vi "Read Format String.vi"(9 "NumericText in":refnum<class "NumericText.lvclass">) -> (3 "NumericText out":refnum<class "NumericText.lvclass">, 4 "Format String":string)   [LabVIEW 2014, in "Raspberry Pi Compatible Compiler for LabVIEW.lvlib" / "NumericText.lvclass"]
uses:
  NumericText.lvclass
  NumericText.lvclass/NumericText.ctl
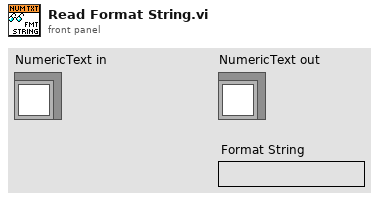
[diagram p1: front panel]
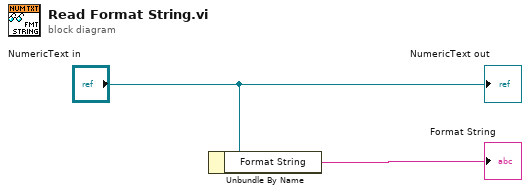
[diagram p0: block diagram]
diagram:
  n1 = Unbundle By Name("NumericText in") -> ("Format String"=→"Format String":string)
  "NumericText out" <- "NumericText in"
